vi "Tx Read Triggers (Pulse Output).vi"(9 "input valid (nc)":bool, 11 "niUSRP Sync":refnum<class "niUSRP Sync v1 FPGA.lvclass">, 12 "ready for output (nc)":bool, 13 "external trigger":bool) -> (8 "future trigger":bool, 10 "output valid":bool, 14 "ready for input (nc)":bool, 15 "niUSRP Sync":refnum<class "niUSRP Sync v1 FPGA.lvclass">)   [LabVIEW 2025, in "niUSRP Sync v1 FPGA.lvclass"]
doc: "this VI handles the processing of triggers and initiates the Aglinment calculation used to align Data with its corresponding Trigger. the calculation takes place before an acquisition is in progress and must be run each time the configuration changes. <b>the calculation should not be run for OTF (on the fly) changes.</b>"
uses:
  niUSRP Sync v1 FPGA.lvclass
  niUSRP Sync v1 FPGA.lvclass/niUSRP Sync v1 FPGA.ctl
  <vilib>/rvi/eio/common/nirviEmuTemplateMethod_errors.vi
  <vilib>/rvi/DataTransferAndStorage/Container/Common/niFpgaContainerExecOnDevCompGetState.vi
  <vilib>/rvi/Emulation/niFpgaEmulationIsFPGAContextNoSignature.vi
  <vilib>/rvi/DataTransferAndStorage/Container/Common/niFpgaContainerGetUniqueNameForEmu.vi
  <vilib>/rvi/Memory/Memory_Emulation/niFpgaMemoryEmulationCacheClearOnFirstRun.vi
  <vilib>/rvi/Memory/Memory_Emulation/nirvimemoryEmulationManagerCache_MakeExclusive.vi
  <vilib>/rvi/Memory/Memory_Emulation/niFpgaMemoryEmulationValidateCache.vi
  <vilib>/rvi/Memory/Memory_Emulation/nirvimemoryEmulationManagerCache_InsertValue.vi
  <vilib>/Utility/error.llb/Clear Errors.vi
  <vilib>/rvi/Memory/Memory_Emulation/nirvimemoryEmulationManagerCache_ReleaseExclusive.vi
  <vilib>/rvi/Memory/Memory_Emulation/nirvimemoryEmulationManagerCache_GetValue.vi
  <vilib>/rvi/Memory/Memory_Emulation/nirvimemoryEmulationManagerCache_SetValue.vi
  <vilib>/rvi/Emulation/niFpgaProcessEmulError.vi
  <vilib>/rvi/Emulation/niFpgaSctlEmulationGetInTimedLoop.vi
  <vilib>/eio/EIONode/EIONode.xnode
  <vilib>/rvi/DataTransferAndStorage/Container/XNode/niFpgaContainer.xnode
  <vilib>/rvi/DataTransferAndStorage/Register/Emulation/niFpgaRegisterEmulationRefIn.vi
  <instrlib>/_niInstr/Basic Elements/v1/FPGA/niInstr Basic Elements v1 FPGA.lvlib
  <instrlib>/niUsrpRio/Time/v1/FPGA/niUsrpRio Time v1 FPGA.lvlib
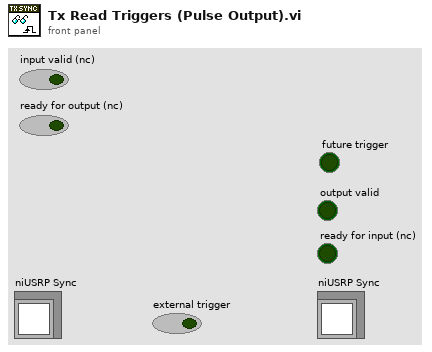
[diagram p1: front panel]
types:
  T1 = enum8{"Software", "Digital Edge", "Rx Start Trigger", "Tx Start Trigger", "Immediate", "Future Time Event"}
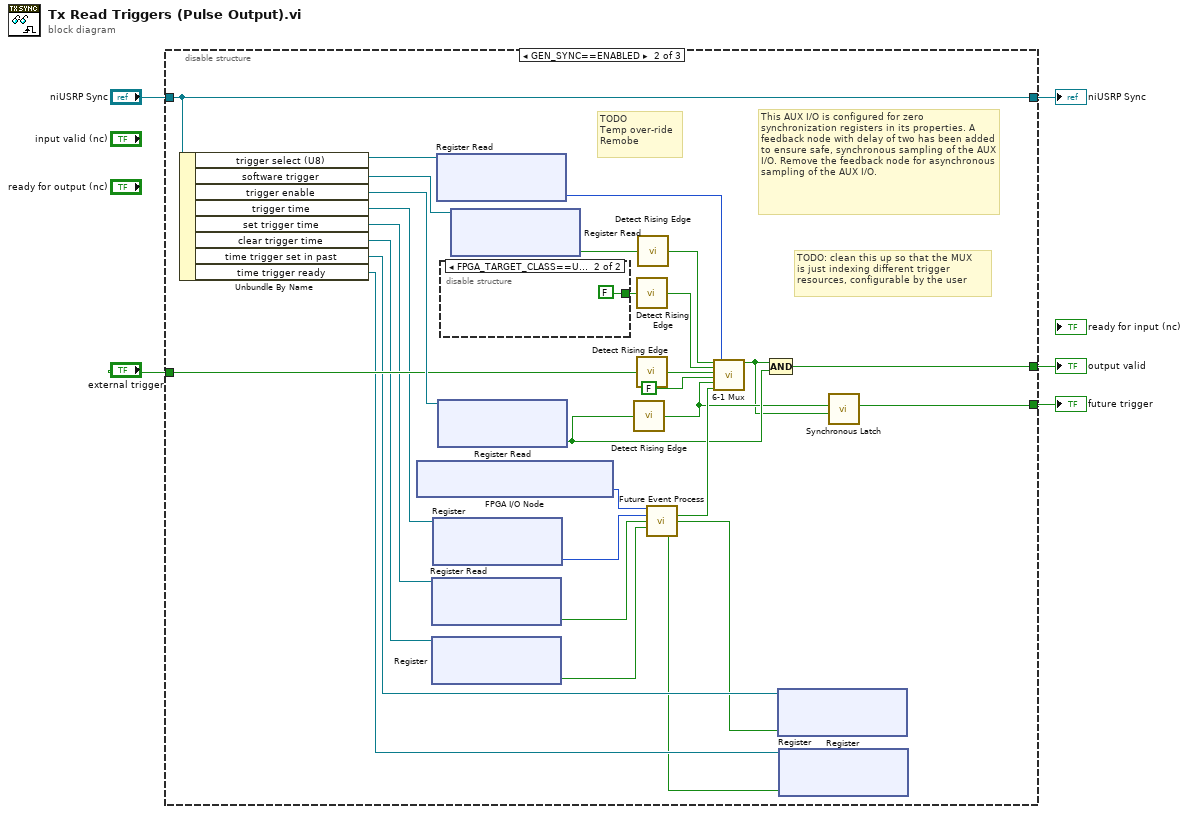
[diagram p0: block diagram]
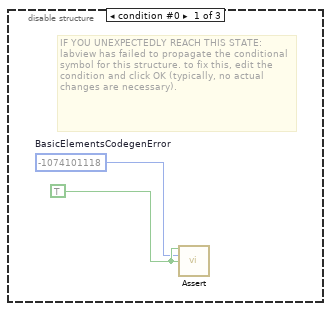
[diagram p2: hidden frame]
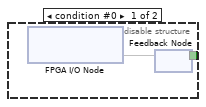
[diagram p3: hidden frame]
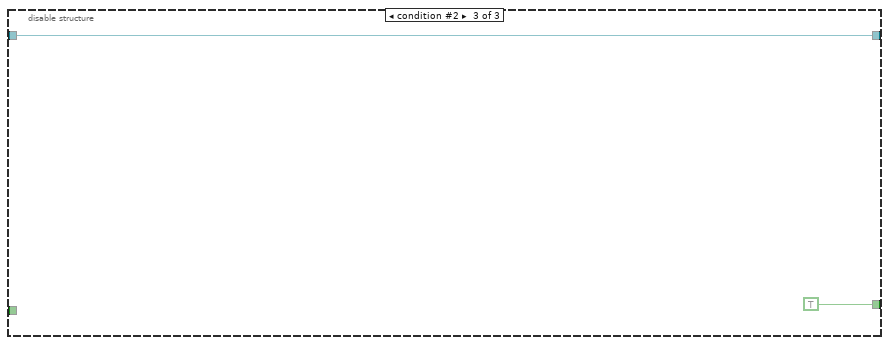
[diagram p4: hidden frame]
diagram:
  n1 = disable-structure shown="GEN_SYNC==ENABLED" {
    disable-tunnel: "niUSRP Sync" -> [_ w29 w41]
    disable-tunnel: [_ w29 w41] -> w4
    disable-tunnel: [_ w28 TRUE] -> w3
    disable-tunnel: "external trigger" -> [_ w26 _]
    disable-tunnel: [_ w9 _] -> w1
    frame condition #0 {
      w7 = TRUE ("assert")
      w6 = -1074101118  # BasicElementsCodegenError
      # "IF YOU UNEXPECTEDLY REACH THIS STATE:\nlabview has failed to propagate the conditional symbol for this structure. to fix this, edit the condition and click OK (typically, no actual changes are necessary)."
      n2 = call <instrlib>:"Assert.vi"("assert"=w7, "error code"=w6, "enable show error"=w7) -> ()  [unwired: 13 in]
    }
    frame condition #1 (active) {
      # "TODO\nTemp over-ride\nRemobe"
      # "TODO: clean this up so that the MUX\nis just indexing different trigger\nresources, configurable by the user"
      # "This AUX I/O is configured for zero synchronization registers in its properties. A feedback node with delay of two has been added to ensure safe, synchronous sampling of the AUX I/O. Remove the feedback node for asynchronous sampling of the AUX I/O."
      n3 = Unbundle By Name(w29) -> ("trigger select (U8)"=w34:refnum<k21>, "software trigger"=w33:refnum<k21>, "trigger enable"=w31:refnum<k21>, "trigger time"=w23:refnum<k21>, "set trigger time"=w20:refnum<k21>, "clear trigger time"=w19:refnum<k21>, "time trigger set in past"=w18:refnum<k21>, "time trigger ready"=w17:refnum<k21>)
      n4 = xnode "FPGA I/O Node"() -> ("Daughterboard 0\\Radio Time"=w22:u64)  [unwired: 1 in, 1 out]
      n5 = xnode "Register Read"("Register In"=w20) -> ("Data"=w12:bool)  [unwired: 1 out]
      n6 = xnode "Register"("Register In"=w19) -> ("Data"=w14:bool)  [unwired: 1 out]
      n7 = xnode "Register"("Register In"=w23) -> ("Data"=w21:u64)  [unwired: 1 out]
      n8 = xnode ("Register Read")("Register In"=w34) -> ("Data"=w24:T1)  [unwired: 1 out]
      n9 = xnode ("Register Read")("Register In"=w31) -> ("Data"=w11:bool)  [unwired: 1 out]
      n10 = disable-structure shown="FPGA_TARGET_CLASS==USRP_X410||FPGA_TARGET_CLASS==USRP_X410__EMBEDDED____UNSUPPORTED" {
        disable-tunnel: [w37 FALSE] -> w27
        frame condition #0 {
          n11 = xnode "FPGA I/O Node"() -> ("AUX I/O 0"=w38)  [unwired: 1 in, 1 out]
          n12 = feedback #1() -> (w37)  [unwired: 1 in]
          n13 = feedback-in #1(w38) -> ()
        }
        frame condition #1 (active) {
        }
      }
      n14 = xnode ("Register Read")("Register In"=w33) -> ("Data"=w32:bool)  [unwired: 1 out]
      n15 = call <instrlib>:"Detect Rising Edge.vi"("signal"=w11) -> ("edge detected"=w10:bool)  [unwired: 14 in]
      n16 = call <instrlib>:"Detect Rising Edge.vi"("signal"=w27) -> ("edge detected"=w35:bool)  [unwired: 14 in]
      n17 = call <instrlib>:"Detect Rising Edge.vi"("signal"=w26) -> ("edge detected"=w25:bool)  [unwired: 14 in]
      n18 = call <instrlib>:"Detect Rising Edge.vi"("signal"=w32) -> ("edge detected"=w36:bool)  [unwired: 14 in]
      n19 = call <instrlib>:"Future Event Process.vi"("time"=w22, "future event.time"=w21, "future event.set"=w12, "future event.clear"=w14) -> ("event.occurred"=w15:bool, "future event.set in past"=w13:bool, "future event.ready"=w16:bool)  [unwired: 8 in, 1 out]
      n20 = call "6-1 Mux.vi"("input 0"=w36, "input 1"=w35, "input 2"=w25, "input 3"=FALSE ("other start trigger"), "input 4"=w10, "input 5"=w15, "select"=w24) -> ("output"=w8:bool)  [unwired: 12 in]
      n21 = Compound Arithmetic op=AND(w8, w11) -> (w28:bool)
      n22 = xnode "Register"("Data"=w13, "Register In"=w18) -> ()  [unwired: 1 out]
      n23 = xnode "Register"("Data"=w16, "Register In"=w17) -> ()  [unwired: 1 out]
      n24 = call <instrlib>:"Synchronous Latch.vi"("clear"=w8, "set"=w10) -> ("out"=w9:bool)  [unwired: 9 in]
    }
    frame condition #2 {
    }
  }
  "output valid" <- w3
  "niUSRP Sync" <- w4
  "future trigger" <- w1
